vi "同步JK触发器（CP下降沿触发）.vi"(1 "k":bool, 2 "c":bool, 3 "J":bool) -> (0 "Q":bool)   [LabVIEW 2012, in "触发器.lvlib"]
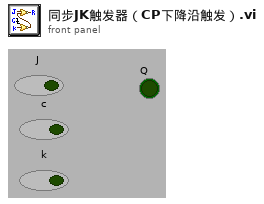
[diagram p1: front panel]
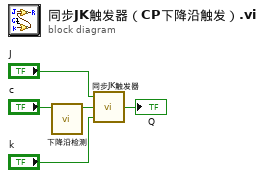
[diagram p0: block diagram]
diagram:
  n1 = call "下降沿检测.vi"("input"="c") -> ("output"=w4:bool)  [unwired: 9 in, 1 out]
  n2 = call "同步JK触发器.vi"("k"="k", "c"=w4, "J"="J") -> ("Q"=→"Q":bool)
